vi "trouble_shoot.vi"() -> ()   [LabVIEW 2021]
panel:
  out "return count":u32
  out "read buffer":string
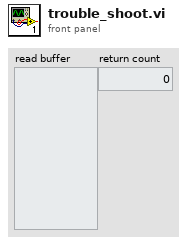
[diagram p1: front panel]
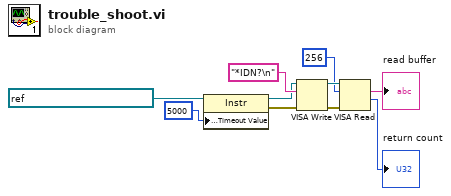
[diagram p0: block diagram]
diagram:
  n1 = property class="Instr"(reference=refnum<visa-resource-name> "GPIB1::5::INSTR" ("VISA resource name"), "General Settings:Timeout Value"=u32 5000) -> (reference out=w2:refnum<visa-resource-name>, error out=w1:errorcluster)  [unwired: 1 in]
  n2 = VISA Write(VISA resource name=w2, write buffer="*IDN?\n", error in (no error)=w1) -> (VISA resource name out=w9:refnum<visa-resource-name>, error out=w5:errorcluster)  [unwired: 1 out]
  n3 = VISA Read(VISA resource name=w9, byte count=u32 256, error in (no error)=w5) -> (read buffer=→"read buffer":string, return count=→"return count":u32)  [unwired: 2 out]
